vi "Fill Zone Special Strings.vi"(10 "JSONCluster in":T1, 11 "value in":string) -> (3 "replaced value":string)   [LabVIEW 2015]
uses:
  Typedef/JSONCluster.ctl
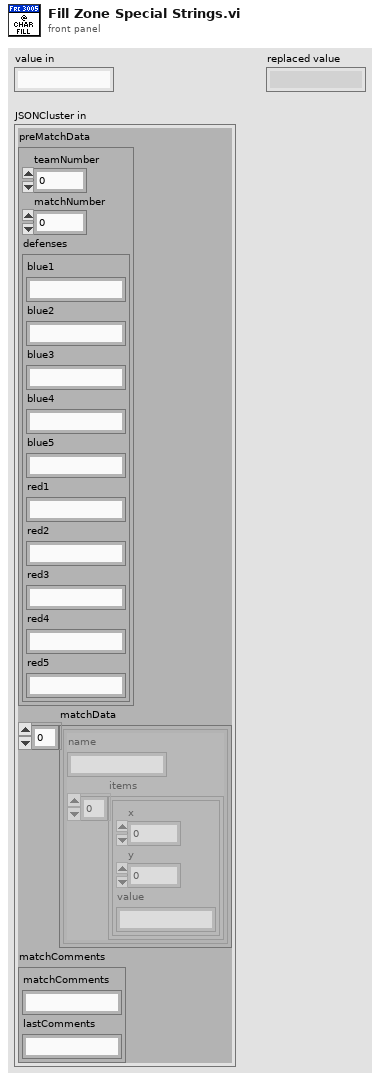
[diagram p1: front panel]
types:
  T1 = typedef "JSONCluster.ctl" = cluster{"preMatchData":cluster{"teamNumber":i32, "matchNumber":i32, "defenses":cluster{"blue1":string, "blue2":string, "blue3":string, "blue4":string, "blue5":string, "red1":string, "red2":string, "red3":string, "red4":string, "red5":string}}, "matchData":cluster{"name":string, "items":cluster{"x":i32, "y":i32, "value":string}[]}[], "matchComments":cluster{"matchComments":string, "lastComments":string}}
  T2 = cluster{"blue1":string, "blue2":string, "blue3":string, "blue4":string, "blue5":string, "red1":string, "red2":string, "red3":string, "red4":string, "red5":string}
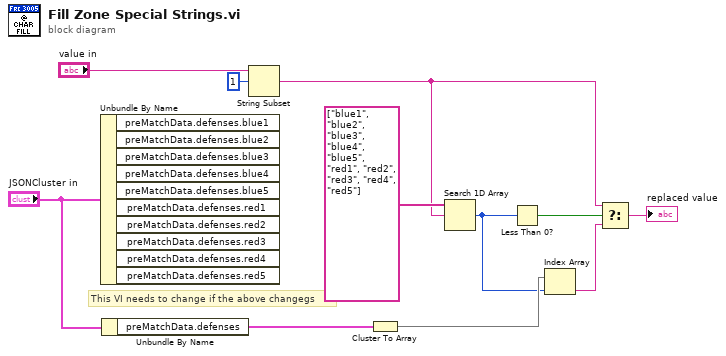
[diagram p0: block diagram]
diagram:
  # "This VI needs to change if the above changegs"
  n1 = Unbundle By Name("JSONCluster in") -> ()  [unwired: 10 out]
  n2 = Unbundle By Name("JSONCluster in") -> ("preMatchData.defenses"=w8:T2)
  n3 = String Subset(string="value in", offset (0)=1) -> (substring=w2:string)  [unwired: 1 in]
  n4 = Cluster To Array(cluster=w8) -> (array=w6:string[])
  n5 = Search 1D Array(1D array=string[] ["blue1", "blue2", "blue3", "blue4", "blue5", "red1", "red2", "red3", "red4", "red5"], element=w2) -> (index of element=w5:i32)  [unwired: 1 in]
  n6 = Less Than 0?(x=w5) -> (x < 0?=w4:bool)
  n7 = Index Array(array=w6, index=w5) -> (element=w3:string)
  n8 = Select(t=w2, s=w4, f=w3) -> (s? t:f=→"replaced value":string)
